vi "Animation.vi"(8 "Error In":errorcluster, 11 "Animation Config":T1) -> (0 "Error Out":errorcluster, 3 "Animation Config":T1)   [LabVIEW 2011, in "LVH-Toolbox.lvlib" / "LVH-SystemTools.lvlib"]
uses:
  LVH-SystemTools.lvlib
  Animation Config.ctl
  <vilib>/picture/picture.llb/imagedata.ctl
  Type Defs/FGV States.ctl
  <vilib>/picture/picture.llb/Draw True-Color Pixmap.vi
panel:
  out "Image":picture
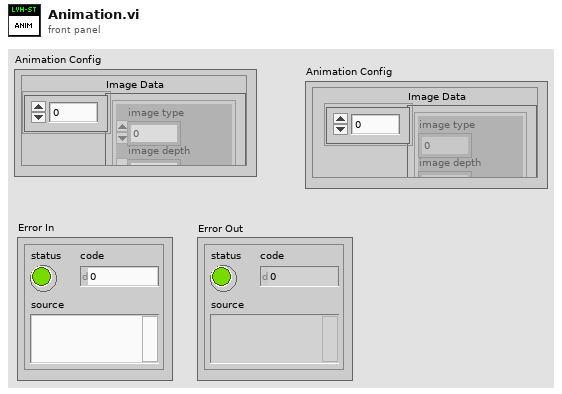
[diagram p1: front panel]
types:
  T1 = typedef "LVH-Toolbox.lvlib/LVH-SystemTools.lvlib/Animation Config.ctl" = cluster{"Image Data":T2[], "FPS":u32, "Position":cluster{"X":i16, "Y":i16}}
  T2 = typedef "imagedata.ctl" = cluster{"image type":i32, "image depth":i32, "image":u8[], "mask":u8[], "colors":u32[], "Rectangle":cluster{"left":i16, "top":i16, "right":i16, "bottom":i16}}
  T3 = typedef "LVH-Toolbox.lvlib/LVH-SystemTools.lvlib/FGV States.ctl" = enum16{"Init", "Set", "Get"}
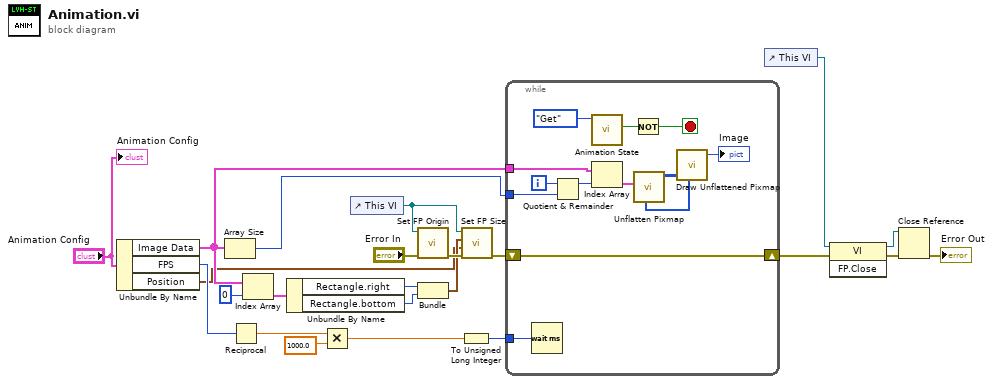
[diagram p0: block diagram]
diagram:
  n1 = Unbundle By Name("Animation Config") -> ("Image Data"=w20:T2[], "FPS"=w15:u32, "Position"=w1:cluster{"X":i16, "Y":i16})
  n2 = Array Size(array=w20) -> (size(s)=w23:i32)
  n3 = Reciprocal(x=w15) -> (1/x=w18:dbl)
  n4 = Index Array(array=w20, index=0) -> (element=w19:T2)
  n5 = Unbundle By Name(w19) -> ("Rectangle.right"=w10:i16, "Rectangle.bottom"=w9:i16)
  n6 = Multiply(x=w18, y=1000.0) -> (x*y=w16:dbl)
  n7 = control-ref of="This VI"() -> (w12:refnum<vi>)
  n8 = call "Set FP Origin.vi"("Error In"="Error In", "VI Ref"=w12) -> ("Error Out"=w11:errorcluster)  [unwired: 9 in]
  n9 = Bundle("right"=w10, "bottom"=w9) -> (w8:cluster{"right":i16, "bottom":i16})  [unwired: 1 in]
  n10 = To Unsigned Long Integer(number=w16) -> (unsigned 32bit integer=w14:u32)
  n11 = call "Set FP Size.vi"("Error In"=w11, "Position"=w1, "Size"=w8, "VI Ref"=w12) -> ("Error Out"=w7:errorcluster)  [unwired: 7 in]
  n12 = while {
    tunnel: w23 -> [w35]
    tunnel: w20 -> [w30]
    shift-right: [w28] -> w2
    shift-left: w7 -> [w28]
    tunnel: w14 -> [w24]
    i -> [w36]
    stop <- w25 stop-if-true
    n13 = Wait (ms)(milliseconds to wait=w24) -> ()  [unwired: 1 out]
    n14 = Quotient & Remainder(x=w36, y=w35) -> (x-y*floor(x/y)=w34:i32)  [unwired: 1 out]
    n15 = call "Animation State.vi"("Function"=FGV_States."Get") -> ("Running?"=w26:bool)  [unwired: 10 in]
    n16 = Index Array(array=w30, index=w34) -> (element=w29:T2)
    n17 = Not(x=w26) -> (.not. x?=w25:bool)
    n18 = call <vilib>:"Unflatten Pixmap.vi"("image data"=w29) -> ("24-bit pixmap"=w32:u32[][], "mask"=w31:u8[])  [unwired: 4 in, 5 out]
    n19 = call-poly <vilib>:"Draw Unflattened Pixmap.vi"("data (RGB format)"=w32, "mask"=w31) -> ("new picture"=→"Image":picture)  [unwired: 7 in]
  }
  n20 = control-ref of="This VI"() -> (w6:refnum<vi>)
  n21 = invoke class="VI" method="FP.Close"(reference=w6, error in=w2) -> (reference out=w5:refnum<vi>, error out=w4:errorcluster)  [unwired: 1 in, 1 out]
  n22 = Close Reference(reference=w5, error in (no error)=w4) -> (error out=→"Error Out":errorcluster)
  "Animation Config" <- "Animation Config"
